vi "Write State.vi"(8 "error in":errorcluster, 10 "State":bool, 11 "Switch in":refnum<class "Switch.lvclass">) -> (0 "error out":errorcluster, 3 "Switch out":refnum<class "Switch.lvclass">)   [LabVIEW 2015, in "Switch.lvclass"]
uses:
  Switch.lvclass
  Switch.lvclass/Switch.ctl
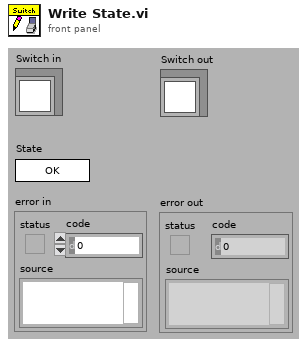
[diagram p1: front panel]
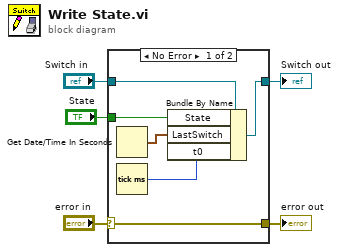
[diagram p0: block diagram]
diagram:
  n1 = case shown="No Error" "error in" {
    selector: "error in" -> [w11 w12]
    tunnel: [w11 w12] -> w4
    tunnel: [w9 w13] -> w2
    tunnel: "Switch in" -> [w10 w13]
    tunnel: "State" -> [w8 _]
    frame No Error {
      n2 = Get Date/Time In Seconds() -> (seconds since 1Jan1904=w7:timestamp)
      n3 = Tick Count (ms)() -> (millisecond timer value=w6:u32)
      n4 = Bundle By Name(cluster=w10, "State"=w8, "LastSwitch"=w7, "t0"=w6) -> (w9:refnum<class "Switch.lvclass">)
    }
    frame Error {
    }
  }
  "error out" <- w4
  "Switch out" <- w2
